vi "Dispose.vi"(8 "error in":errorcluster, 11 "ChicagoStylePepperoniPizza":refnum<class "ChicagoStylePepperoniPizza.lvclass">) -> (0 "error out":errorcluster)   [LabVIEW 2020, in "FactoryMethod.lvlib" / "PizzaFactoryMethod.lvlib" / "ChicagoStylePepperoniPizza.lvclass"]
uses:
  ChicagoStylePepperoniPizza.lvclass
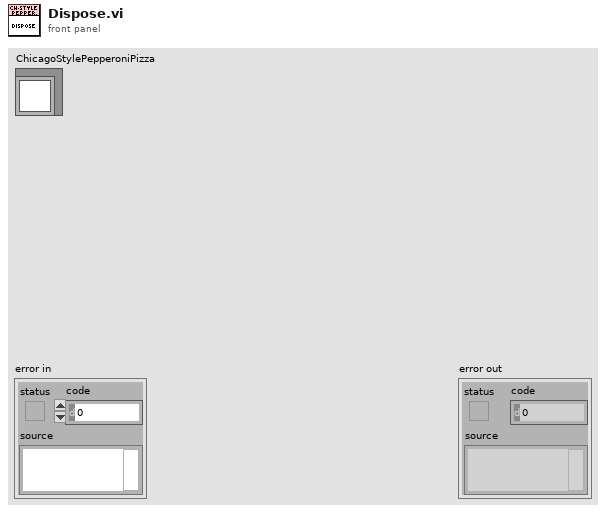
[diagram p1: front panel]
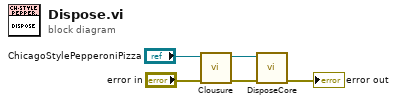
[diagram p0: block diagram]
diagram:
  n1 = call-dynamic "Clousure.vi"("error in"="error in", "ChicagoStylePepperoniPizza"="ChicagoStylePepperoniPizza") -> ("error out"=w3:errorcluster, "ChicagoStylePepperoniPizza"=w4:refnum<class "ChicagoStylePepperoniPizza.lvclass">)  [unwired: 8 in]
  n2 = call-dynamic "DisposeCore.vi"("error in (no error)"=w3, "ChicagoStylePepperoniPizza"=w4) -> ("error out"=→"error out":errorcluster)  [unwired: 8 in, 1 out]
